vi "Complex Compact Cho Matrix Inverse.vi"(0 "Cholesky  Compact Array":cluster{"Compact Array":cdb[], "array type":i32} {"array type" items=["lower triangular", "upper triangular"]; "Compact Array" format="%.2f"}) -> (1 "Inverse Array":cluster{"Compact Array":cdb[], "array type":i32} {"array type" items=["lower triangular", "upper triangular"]; "Compact Array" format="%.2f"}, 2 "error":i32)   [LabVIEW 2014, in "NI_AALBase.lvlib"]
doc: "Solves a linear system of simultaneous equations, if possible. The system is solved using the method known as L-U decomposition."
uses:
  NI_AALBase.lvlib
  lvanlys.dll
panel:
  # "Complex Compact Cho Matrix Inverse"
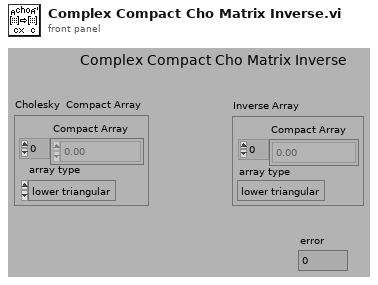
[diagram p1: front panel]
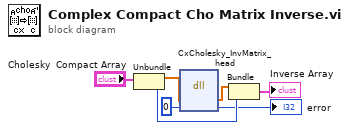
[diagram p0: block diagram]
diagram:
  n1 = Unbundle("Cholesky  Compact Array") -> ("Compact Array"=w4:cdb[], "array type"=w5:i32)
  n2 = dll-call lib="C:/Program Files (x86)/National Instruments/LabVIEW 2014/resource/lvanlys.*" fn="CxCholesky_InvMatrix_head"("Compact Array"=w4, 0) -> ("Compact Array"=w3:cdb[], →"error":i32)  [unwired: 4 in, 2 out]
  n3 = Bundle("Compact Array"=w3, "array type"=w5) -> (→"Inverse Array":cluster{"Compact Array":cdb[], "array type":i32})  [unwired: 1 in]
